vi "Autonomous.vi"() -> ()   [LabVIEW 2023]
doc: "This VI starts when autonomous period begins, and will automatically be terminated when it ends. You can carry out timed or sensor driven operations directly to I/O or to subsystems without needing to return to the caller."
uses:
  Drive/Implementation/Drive Operations.ctl
  Support Code/Teleop Util/Coral States.ctl
  Support Code/Teleop Util/Scoring Levels.ctl
  Coral/Implementation/Coral Operations.ctl
  <vilib>/Rock Robotics/WPI/Utilities/WPI_GetSetVariantRefNum.vi
  Framework/Robot Global Data.vi
  <vilib>/Rock Robotics/Network Tables/NT Read String.vi
  <vilib>/Rock Robotics/Network Tables/NT Read String Array.vi
  <vilib>/Utility/file.llb/Read Delimited Spreadsheet (string).vi
panel:
  in  "Is Blue Alliance? 2":bool=TRUE
  in  "Is Blue Alliance?":bool=TRUE
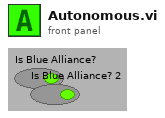
[diagram p1: front panel]
types:
  T1 = typedef "WPI_JoystickDevRef.ctl" = cluster{"Device":T2}
  T2 = typedef "WPI_JoystickDeviceEnum.ctl" = enum16{"USB 0", "USB 1", "USB 2", "USB 3", "USB 4", "USB 5"}
  T3 = typedef "Coral Operations.ctl" = enum16{"Reserve", "Read Current", "Immediate", "Calibrate"}
  T4 = typedef "Scoring Levels.ctl" = enum16{"Trough", "L2", "L3", "L4", "Default"}
  T5 = typedef "Coral States.ctl" = enum16{"Grounded", "Coral Intake", "Scoring Sequence", "Hold Position", "Score", "Manual Override", "Climb Safety Mode"}
  T6 = typedef "Drive Operations.ctl" = enum16{"Reserve", "Read Current", "Immediate", "Calibrate", "Reef Align", "Auto"}
  T7 = cluster{dbl, "Command out":cluster{"Name":string, "vi reference":refnum<vi>, i32[], variant[]}}[]
  T8 = typedef "Robot Velocities.ctl" = cluster{"X Velocity":dbl, "Y Velocity":dbl, "Rotational \nVelocity":dbl}
  T9 = typedef "CTRE_PigeonIMU_DeviceRef.ctl" = cluster{"DeviceStatus":errorcluster, "Device Number":u8, "Type":T10, "Device ID":u32, "Handle":u64, "UsageFrame":u32, "Library Path":path}
  T10 = typedef "CTRE_PigeonIMU_ConnectionType.ctl" = u32
  T11 = cluster{"Velocities":T8[], "Positions":cluster{"x":dbl, "y":dbl, "th":dbl}[], cluster{dbl, "Command out":cluster{"Name":string, "vi reference":refnum<vi>, i32[], variant[]}}[], "Zero Velocity?":bool[]}
  T12 = typedef "Command Status Info.ctl" = cluster{"Name":string, "Status":T13, "notifier out":T14}
  T13 = typedef "Completion Status.ctl" = enum16{"Successful", "Aborted", "Incomplete"}
  T14 = typedef "Completion Notifier.ctl" = refnum<notifier>
  T15 = cluster{"Trough":dbl, "L2":dbl, "L3":dbl, "L4":dbl}
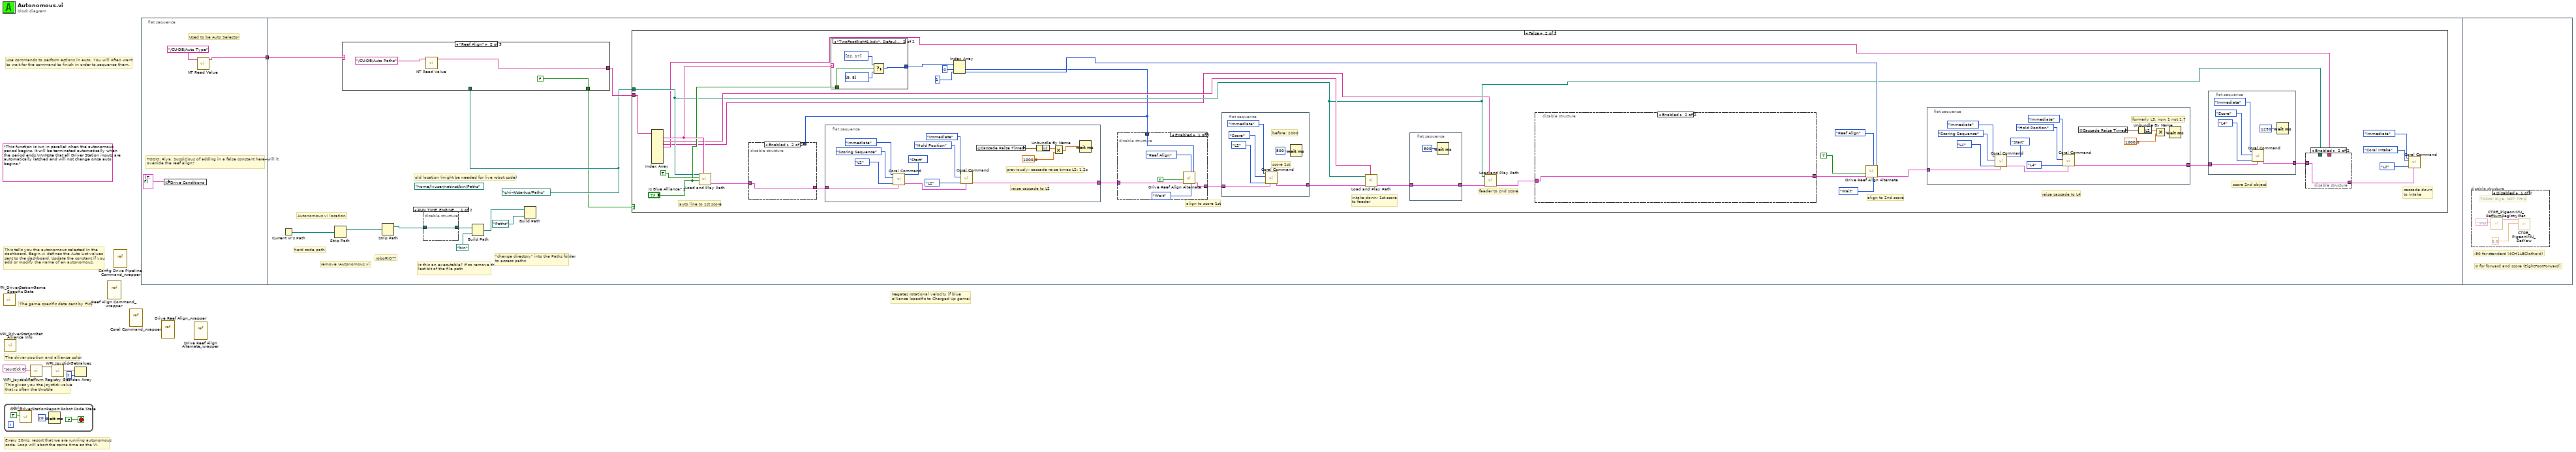
[diagram p0: block diagram]
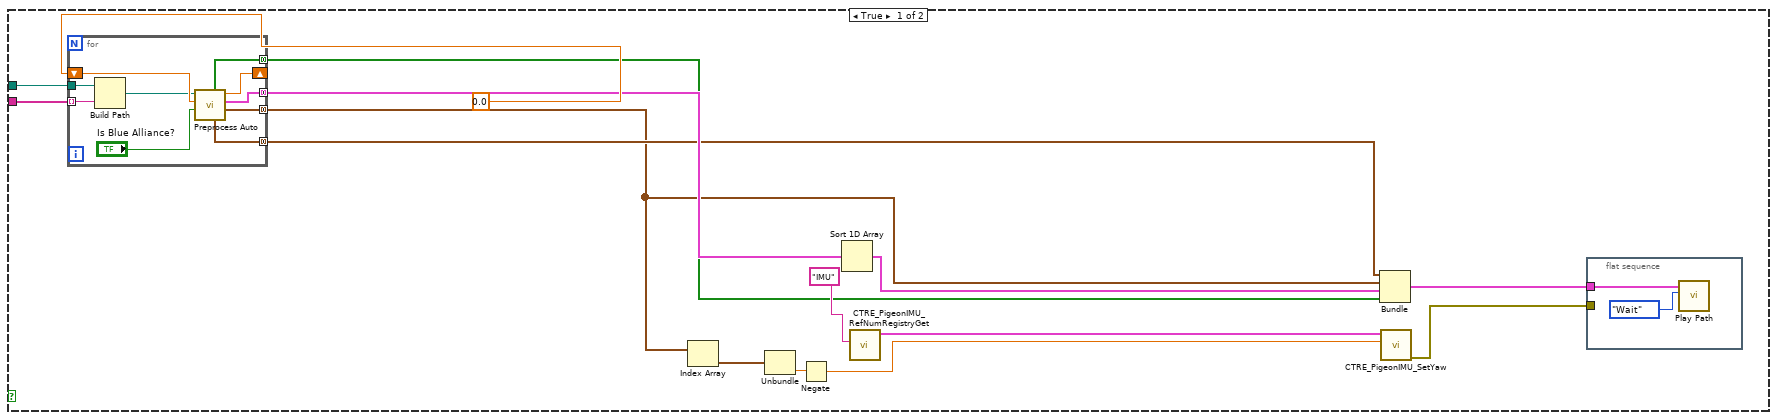
[diagram p2: hidden frame]
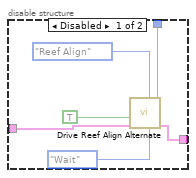
[diagram p3: hidden frame]
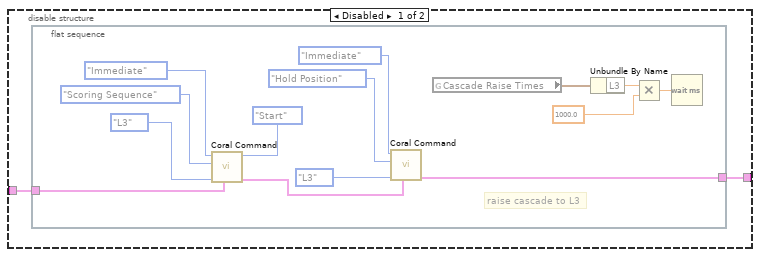
[diagram p5: hidden frame]
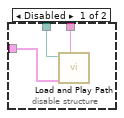
[diagram p6: hidden frame]
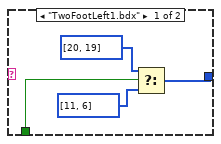
[diagram p7: hidden frame]
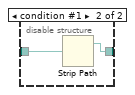
[diagram p8: hidden frame]
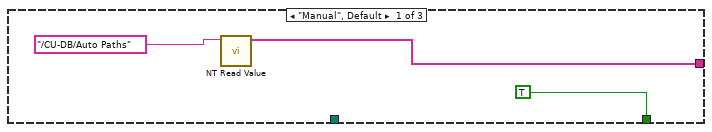
[diagram p9: hidden frame]
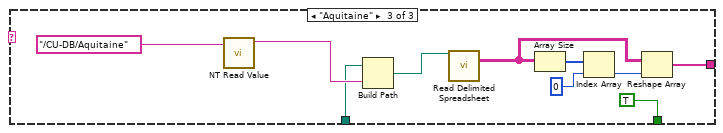
[diagram p10: hidden frame]
diagram:
  (unwired) "This function is run in parallel when the autonomous period begins. It will be terminated automatically when the period ends.\n\nNote that all Driver Station inputs are automatically latched and will not change once auto begins."
  # "Negates rotational velocity if blue alliance (specific to Charged Up game)"
  # "The game specific data sent by FMS"
  # "This tells you the autonomous selected in the \ndashboard. Begin.vi defines the Auto List values\nsent to the dashboard. Update the constant if you\nadd or modify the name of an autonomous."
  # "Every 20ms, report that we are running autonomous\ncode. Loop will abort the same time as the VI."
  # "This gives you the joystick value\nthat is often the throttle"
  # "Use commands to perform actions in auto. You will often want\nto wait for the command to finish in order to sequence them."
  # "The driver position and alliance color"
  n1 = call <vilib>:"WPI_DriverStationGame Specific Data.vi"() -> ()  [unwired: 11 in, 1 out]
  n2 = while {
    stop <- FALSE stop-if-true
    n3 = call <vilib>:"WPI_DriverStationReport Robot Code State.vi"("Autonomous"=TRUE) -> ()  [unwired: 10 in, 1 out]
    n4 = Wait (ms)(milliseconds to wait=u32 20) -> ()  [unwired: 1 out]
  }
  n5 = call <vilib>:"WPI_DriverStationGet Alliance Info.vi"() -> ()  [unwired: 12 out]
  n6 = call <vilib>:"WPI_JoystickRefNum Registry Get.vi"("refnum name"="Joystick 0") -> ("JoystickDevRef"=w4:T1)  [unwired: 1 in, 9 out]
  n7 = call <vilib>:"WPI_JoystickGetValues.vi"("JoystickDevRef"=w4) -> ("Axes"=w3:dbl[])  [unwired: 6 in, 4 out]
  n8 = Index Array(array=w3, index=2) -> ()  [unwired: 1 out]
  n9 = vi-ref "Reef Align Command_wrapper.vi"() -> ()  [unwired: 1 out]
  n10 = vi-ref "Config Drive Pipeline Command_wrapper.vi"() -> ()  [unwired: 1 out]
  n11 = vi-ref "Coral Command_wrapper.vi"() -> ()  [unwired: 1 out]
  n12 = flat-sequence {
    tunnel: [w9] -> w1
    tunnel: w1 -> [w13]
    frame #0 {
      # "Used to be Auto Selector"
      # "TODO: Riya. Suspicious of adding in a false constant here--will it override the reef align?"
      n13 = global write "Robot Global Data.vi" "Drive Conditions"(cluster{"Field Centric":bool, bool} {"Field Centric"=TRUE, FALSE} ("Drive Conditions")) -> ()
      n14 = call-poly <vilib>:"NT Read Value.vi"("name"="/CU-DB/Auto Type") -> ("value"=w9:string)  [unwired: 8 in, 2 out]
    }
    frame #1 {
      (unwired) path "/home/lvuser/natinst/bin/Paths"
      w14 = path "c:/ni-rt/startup/Paths"
      # "old location (might be needed for live robot code)"
      # "\"change directory\" into the Paths folder to access paths"
      # "is this an executable? if so remove that last bit of the file path"
      # "roboRIO??"
      # "remove \\Autonomous.vi"
      # "Autonomous.vi location"
      # "hard code path"
      n15 = Current VI's Path() -> (path=w19:path)
      n16 = Strip Path(path=w19) -> (stripped path=w20:path)  [unwired: 1 out]
      n17 = case shown="\"Reef Align\"" w13 {
        tunnel: w14 -> [_ _ w183]
        tunnel: [w171 w174 w177] -> w17
        tunnel: [TRUE FALSE TRUE ("Boolean")] -> w12
        frame "Manual", Default {
          n18 = call-poly <vilib>:"NT Read Value.vi"("name"="/CU-DB/Auto Paths") -> ("value"=w171:string[])  [unwired: 8 in, 2 out]
        }
        frame "Reef Align" {
          n19 = call-poly <vilib>:"NT Read Value.vi"("name"="/CU-DB/Auto Paths") -> ("value"=w174:string[])  [unwired: 8 in, 2 out]
        }
        frame "Aquitaine" {
          n20 = call-poly <vilib>:"NT Read Value.vi"("name"="/CU-DB/Aquitaine") -> ("value"=w184:string)  [unwired: 8 in, 2 out]
          n21 = Build Path(base path=w183, name or relative path=w184) -> (appended path=w182:path)
          n22 = call-poly <vilib>:"Read Delimited Spreadsheet.vi"("file path (dialog if empty)"=w182) -> ("all rows"=w178:string[][])  [unwired: 9 in, 5 out]
          n23 = Array Size(array=w178) -> (size(s)=w181:i32[])
          n24 = Index Array(array=w181, index=0) -> (element=w179:i32)
          n25 = Reshape Array(w178, w179) -> (w177:string[])
        }
      }
      n26 = Strip Path(path=w20) -> (stripped path=w22:path)  [unwired: 1 out]
      n27 = disable-structure shown="RUN_TIME_ENGINE==False" {
        disable-tunnel: [w167 w168] -> w21
        disable-tunnel: w22 -> [w167 w169]
        frame condition #0 (active) {
        }
        frame condition #1 {
          n28 = Strip Path(path=w169) -> (stripped path=w168:path)  [unwired: 1 out]
        }
      }
      n29 = Build Path(base path=w21, name or relative path=path "bin") -> (appended path=w15:path)
      n30 = Build Path(base path=w15, name or relative path=path "Paths") -> ()  [unwired: 1 out]
      n31 = case shown="False" w12 {
        tunnel: w17 -> [w26 w80]
        tunnel: w14 -> [w25 w61]
        frame True {
          n32 = for {
            tunnel: [w44] -> w28 mode=concatenating
            tunnel: [w45] -> w27 mode=concatenating
            shift-right: [w49] -> _
            shift-left: 0.0 -> [w47]
            tunnel: [w48] -> w34 mode=concatenating
            tunnel: [w43] -> w29 mode=concatenating
            tunnel: w25 -> [w40]
            tunnel: w26 -> [w41] mode=indexing
            n33 = Build Path(base path=w40, name or relative path=w41) -> (appended path=w42:path)
            n34 = call "Preprocess Auto.vi"("Is Blue Alliance?"="Is Blue Alliance?", "Start Time"=w47, "appended path"=w42) -> ("Positions"=w45:cluster{"x":dbl, "y":dbl, "th":dbl}[], "Array"=w48:T7, "Finish Time"=w49:dbl, "Velocities"=w44:T8[], "Zero Velocity?"=w43:bool[])  [unwired: 4 in]
          }
          n35 = Index Array(array=w27) -> (element=w33:cluster{"x":dbl, "y":dbl, "th":dbl})  [unwired: 1 in]
          n36 = Unbundle(w33) -> ("th"=w32:dbl)  [unwired: 2 out]
          n37 = Negate(x=w32) -> (-x=w31:dbl)
          n38 = Sort 1D Array(array=w34) -> (sorted array=w30:T7)
          n39 = call <vilib>:"CTRE_PigeonIMU_RefNumRegistryGet.vi"("refnum name"="IMU") -> ("PigeonIMUDevRef"=w37:T9)  [unwired: 9 in, 1 out]
          n40 = Bundle("Velocities"=w28, "Positions"=w27, w30, "Zero Velocity?"=w29) -> (w24:T11)  [unwired: 1 in]
          n41 = call <vilib>:"CTRE_PigeonIMU_SetYaw.vi"("Value"=w31, "PigeonIMUDevRef"=w37) -> ("error out"=w23:errorcluster)  [unwired: 8 in, 1 out]
          n42 = flat-sequence {
            tunnel: w24 -> [w38]
            tunnel: w23 -> [_]
            frame #0 {
              n43 = call "Play Path.vi"("Synchronization"=enum16{"Start", "Wait"}."Wait", "Auto Data"=w38) -> ()  [unwired: 9 in, 1 out]
            }
          }
        }
        frame False {
          # "cascade down\nto intake"
          # "score 2nd object"
          # "raise cascade to L4"
          # "align to 2nd score"
          # "feeder to 2nd score"
          # "intake down; 1st score\nto feeder"
          # "align to score 1st"
          # "auto line to 1st score"
          n44 = Index Array(array=w80) -> (element #1=w77:string, element #2=w73:string, element #3=w50:string, element #4=w60:string)  [unwired: 9 in, 5 out]
          n45 = call "Load and Play Path.vi"("filename"=w77, "Is Blue Alliance? in"="Is Blue Alliance? 2", "Set IMU?"=TRUE, "Path"=w61) -> ("Command Info Out"=w53:T12)  [unwired: 6 in]
          n46 = flat-sequence {
            tunnel: w52 -> [w158]
            tunnel: [w155] -> w79
            frame #0 {
              # "previously: cascade raise times L2: 1.2s"
              # "raise cascade to L2"
              n47 = call "Coral Command.vi"("Synchronization"=enum16{"Start", "Wait"}."Start", "Command Info In"=w158, "Setpoint State"=Scoring_Levels."L2", "Coral States"=Coral_States."Scoring Sequence", "Operation"=Coral_Operations."Immediate") -> ("Command Info Out"=w156:T12)  [unwired: 5 in]
              n48 = call "Coral Command.vi"("Command Info In"=w156, "Setpoint State"=Scoring_Levels."L2", "Coral States"=Coral_States."Hold Position", "Operation"=Coral_Operations."Immediate") -> ("Command Info Out"=w155:T12)  [unwired: 6 in]
              n49 = global read "Robot Global Data.vi" "Cascade Raise Times"() -> (w148:T15)
              n50 = Unbundle By Name(w148) -> ("L2"=w147:dbl)
              n51 = Multiply(x=w147, y=1000.0) -> (x*y=w146:dbl)
              n52 = Wait (ms)(milliseconds to wait=w146) -> ()  [unwired: 1 out]
            }
          }
          n53 = case shown="\"TwoFootRight1.bdx\", Default" w77 {
            tunnel: "Is Blue Alliance? 2" -> [w160 w164]
            tunnel: [w161 w163] -> w75
            frame "TwoFootLeft1.bdx" {
              n54 = Select(t=i32[] [20, 19], s=w160, f=i32[] [11, 6]) -> (s? t:f=w161:i32[])
            }
            frame "TwoFootRight1.bdx", Default {
              n55 = Select(t=i32[] [22, 17], s=w164, f=i32[] [9, 8]) -> (s? t:f=w163:i32[])
            }
          }
          n56 = Index Array(array=w75, index #1=0 ("index"), index #2=1 ("index")) -> (element #1=w51:i32, element #2=w64:i32)
          n57 = disable-structure shown="Enabled" {
            disable-tunnel: w53 -> [w84 w88]
            disable-tunnel: [w83 w88] -> w52
            disable-tunnel: w51 -> [w82 _]
            frame Disabled {
              n58 = call "Drive Reef Align Alternate.vi"("Tag ID"=w82, "Synchronication"=enum16{"Start", "Wait"}."Wait", "Operation"=Drive_Operations."Reef Align", "Command Info In"=w84, "Angle Align"=TRUE) -> ("Command Info Out"=w83:T12)  [unwired: 6 in]
            }
            frame Enabled {
            }
          }
          n59 = disable-structure shown="Enabled" {
            disable-tunnel: w79 -> [w94 w95]
            disable-tunnel: [w90 w95] -> w78
            disable-tunnel: w51 -> [w89 _]
            frame Enabled {
              n60 = call "Drive Reef Align Alternate.vi"("Tag ID"=w89, "Synchronication"=enum16{"Start", "Wait"}."Wait", "Operation"=Drive_Operations."Reef Align", "Command Info In"=w94, "Angle Align"=TRUE) -> ("Command Info Out"=w90:T12)  [unwired: 6 in]
            }
            frame Disabled {
            }
          }
          n61 = flat-sequence {
            tunnel: w78 -> [w144]
            tunnel: [w139] -> w72
            frame #0 {
              # "before: 2000"
              # "score 1st"
              n62 = call "Coral Command.vi"("Command Info In"=w144, "Setpoint State"=Scoring_Levels."L2", "Coral States"=Coral_States."Score", "Operation"=Coral_Operations."Immediate") -> ("Command Info Out"=w139:T12)  [unwired: 6 in]
              n63 = Wait (ms)(milliseconds to wait=u32 500) -> ()  [unwired: 1 out]
            }
          }
          n64 = call "Load and Play Path.vi"("filename"=w73, "Command Info In"=w72, "Path"=w61) -> ("Command Info Out"=w71:T12)  [unwired: 7 in]
          n65 = flat-sequence {
            tunnel: w71 -> [w137]
            tunnel: [w137] -> w70
            frame #0 {
              n66 = Wait (ms)(milliseconds to wait=u32 500) -> ()  [unwired: 1 out]
            }
          }
          n67 = call "Load and Play Path.vi"("filename"=w50, "Command Info In"=w70, "Path"=w61) -> ("Command Info Out"=w69:T12)  [unwired: 7 in]
          n68 = disable-structure shown="Enabled" {
            disable-tunnel: w69 -> [w97 w112]
            disable-tunnel: [w96 w112] -> w67
            frame Disabled {
              n69 = flat-sequence {
                tunnel: w97 -> [w111]
                tunnel: [w108] -> w96
                frame #0 {
                  # "raise cascade to L3"
                  n70 = call "Coral Command.vi"("Synchronization"=enum16{"Start", "Wait"}."Start", "Command Info In"=w111, "Setpoint State"=Scoring_Levels."L3", "Coral States"=Coral_States."Scoring Sequence", "Operation"=Coral_Operations."Immediate") -> ("Command Info Out"=w109:T12)  [unwired: 5 in]
                  n71 = call "Coral Command.vi"("Command Info In"=w109, "Setpoint State"=Scoring_Levels."L3", "Coral States"=Coral_States."Hold Position", "Operation"=Coral_Operations."Immediate") -> ("Command Info Out"=w108:T12)  [unwired: 6 in]
                  n72 = global read "Robot Global Data.vi" "Cascade Raise Times"() -> (w101:T15)
                  n73 = Unbundle By Name(w101) -> ("L3"=w100:dbl)
                  n74 = Multiply(x=w100, y=1000.0) -> (x*y=w99:dbl)
                  n75 = Wait (ms)(milliseconds to wait=w99) -> ()  [unwired: 1 out]
                }
              }
            }
            frame Enabled {
            }
          }
          n76 = call "Drive Reef Align Alternate.vi"("Tag ID"=w64, "Synchronication"=enum16{"Start", "Wait"}."Wait", "Operation"=Drive_Operations."Reef Align", "Command Info In"=w67, "Angle Align"=TRUE) -> ("Command Info Out"=w55:T12)  [unwired: 6 in]
          n77 = flat-sequence {
            tunnel: w55 -> [w126]
            tunnel: [w123] -> w54
            frame #0 {
              # "formerly L3, now 1 not 1.7"
              n78 = call "Coral Command.vi"("Synchronization"=enum16{"Start", "Wait"}."Start", "Command Info In"=w126, "Setpoint State"=Scoring_Levels."L4", "Coral States"=Coral_States."Scoring Sequence", "Operation"=Coral_Operations."Immediate") -> ("Command Info Out"=w124:T12)  [unwired: 5 in]
              n79 = call "Coral Command.vi"("Command Info In"=w124, "Setpoint State"=Scoring_Levels."L4", "Coral States"=Coral_States."Hold Position", "Operation"=Coral_Operations."Immediate") -> ("Command Info Out"=w123:T12)  [unwired: 6 in]
              n80 = global read "Robot Global Data.vi" "Cascade Raise Times"() -> (w116:T15)
              n81 = Unbundle By Name(w116) -> ("L2"=w115:dbl)
              n82 = Multiply(x=w115, y=1000.0) -> (x*y=w114:dbl)
              n83 = Wait (ms)(milliseconds to wait=w114) -> ()  [unwired: 1 out]
            }
          }
          n84 = flat-sequence {
            tunnel: w54 -> [w136]
            tunnel: [w131] -> w62
            frame #0 {
              n85 = call "Coral Command.vi"("Command Info In"=w136, "Setpoint State"=Scoring_Levels."L4", "Coral States"=Coral_States."Score", "Operation"=Coral_Operations."Immediate") -> ("Command Info Out"=w131:T12)  [unwired: 6 in]
              n86 = Wait (ms)(milliseconds to wait=u32 1250) -> ()  [unwired: 1 out]
            }
          }
          n87 = disable-structure shown="Enabled" {
            disable-tunnel: w62 -> [w129 w130]
            disable-tunnel: w61 -> [w128 _]
            disable-tunnel: w60 -> [w127 _]
            disable-tunnel: [_ w130] -> w56
            frame Disabled {
              n88 = call "Load and Play Path.vi"("filename"=w127, "Command Info In"=w129, "Path"=w128) -> ()  [unwired: 7 in, 1 out]
            }
            frame Enabled {
            }
          }
          n89 = call "Coral Command.vi"("Command Info In"=w56, "Setpoint State"=Scoring_Levels."L2", "Coral States"=Coral_States."Coral Intake", "Operation"=Coral_Operations."Immediate") -> ()  [unwired: 6 in, 1 out]
        }
      }
    }
    frame #2 {
      # "0 for forward and score (EightFootForward)"
      # "-90 for standard (4CH1LBClothoid)"
      n90 = disable-structure shown="Disabled" {
        frame Disabled {
          # "TODO: Riya. NOT THIS"
          n91 = call <vilib>:"CTRE_PigeonIMU_RefNumRegistryGet.vi"("refnum name"="IMU") -> ("PigeonIMUDevRef"=w186:T9)  [unwired: 9 in, 1 out]
          n92 = call <vilib>:"CTRE_PigeonIMU_SetYaw.vi"("Value"=0.0, "PigeonIMUDevRef"=w186) -> ()  [unwired: 8 in, 2 out]
        }
        frame Enabled {
        }
      }
    }
  }
  n93 = vi-ref "Drive Reef Align_wrapper.vi"() -> ()  [unwired: 1 out]
  n94 = vi-ref "Drive Reef Align Alternate_wrapper.vi"() -> ()  [unwired: 1 out]
